vi "Actor Core.vi"(8 "error in":errorcluster, 11 "CS++DSCAlarmViewer in":refnum<class "CS++DSCAlarmViewer.lvclass">) -> (0 "error out":errorcluster, 3 "Actor out":refnum<class "Actor.lvclass">)   [LabVIEW 2013, in "CS++DSCAlarmViewer.lvlib" / "CS++DSCAlarmViewer.lvclass"]
doc: "(<B>Filename</B>: Actor Framework.lvlib:Actor.lvclass:Actor Core.vi)\n\nReceives messages to the actor, reacts to them, and initiates any error handling that may shut the actor down.\n\nDescendant classes may override this VI to append parallel tasks for the actor to complete while it handles messages. Overrides use the Call Parent Method node."
uses:
  CS++DSCAlarmViewer.lvclass
  <vilib>/ActorFramework/Actor/Actor.lvclass
  CS++DSCAlarmViewer.lvclass/CS++DSCAlarmViewer.ctl
  Core/Actors/CS++GUIActor/CS++GUIActor.lvclass/CS++GUIActor.ctl
  Core/Actors/CS++BaseActor/CS++BaseActor.lvclass/CS++BaseActor.ctl
  Core/Actors/CS++GUIActor/CS++GUIActor.lvclass
  <vilib>/ActorFramework/Actor/Actor.lvclass/Actor.ctl
  <vilib>/ActorFramework/Message Enqueuer/Message Enqueuer.lvclass/Message Enqueuer.ctl
  <vilib>/ActorFramework/Message Enqueuer/Init from Existing Queue.vi
  <vilib>/ActorFramework/Message Enqueuer/Enqueue.vi
  <vilib>/ActorFramework/Message Priority Queue/Priority Enqueue.vi
  <vilib>/ActorFramework/Message Enqueuer/Message Enqueuer.lvclass
  <vilib>/ActorFramework/Stop Msg/Stop Msg.lvclass
  Core/Actors/CS++BaseActor/CS++BaseActor.lvclass
panel:
  in  "Alarm and Event Display":refnum<k7>(container)
  in  "Stop Button":bool
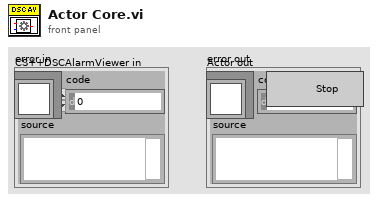
[diagram p1: front panel]
types:
  T1 = enum32{"Invalid", "Standard", "Closed", "Hidden", "Minimized", "Maximized"}
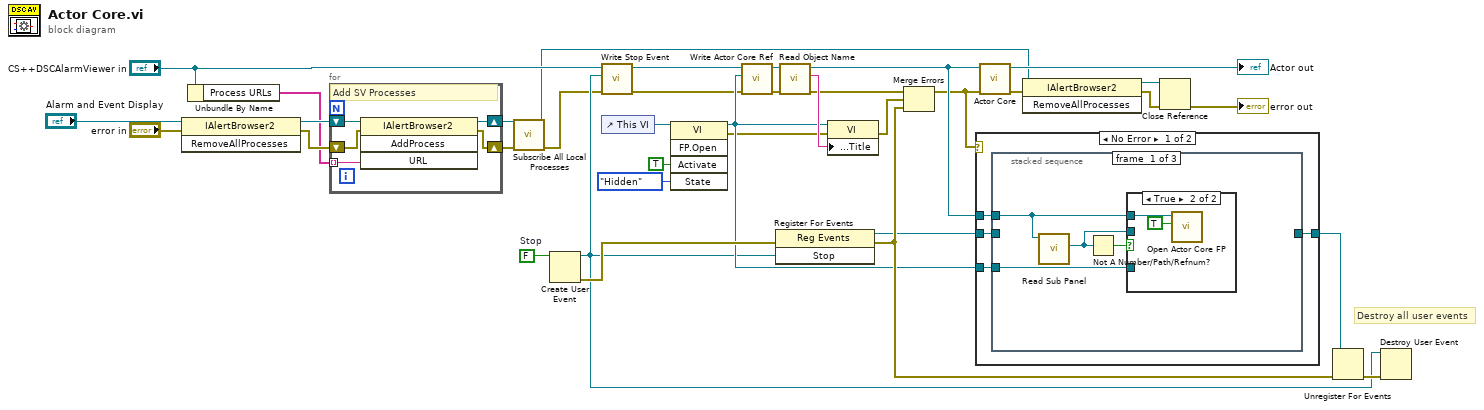
[diagram p0: block diagram]
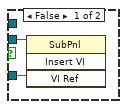
[diagram p2: hidden frame]
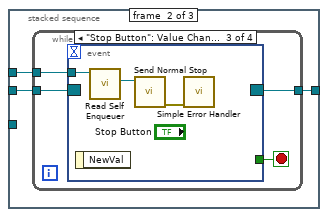
[diagram p3: hidden frame]
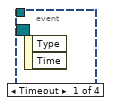
[diagram p4: hidden frame]
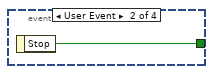
[diagram p5: hidden frame]
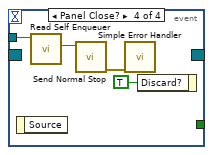
[diagram p6: hidden frame]
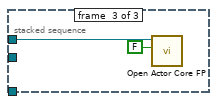
[diagram p7: hidden frame]
diagram:
  w31 = FALSE  # Stop
  # "Destroy all user events"
  n1 = invoke class="IAlertBrowser2" method="RemoveAllProcesses"(reference="Alarm and Event Display", error in="error in") -> (reference out=w14:refnum<k7>, error out=w12:errorcluster)  [unwired: 1 in, 1 out]
  n2 = Unbundle By Name("CS++DSCAlarmViewer in") -> ("Process URLs"=w9:string[])
  n3 = for {
    tunnel: w9 -> [w37] mode=indexing
    shift-right: [w40] -> w13
    shift-left: w14 -> [w41]
    shift-right: [w38] -> w11
    shift-left: w12 -> [w39]
    # "Add SV Processes"
    n4 = invoke class="IAlertBrowser2" method="AddProcess"(reference=w41, error in=w39, "URL"=w37) -> (reference out=w40:refnum<k7>, error out=w38:errorcluster)  [unwired: 1 in, 2 out]
  }
  n5 = call <vilib>:"Subscribe All Local Processes.vi"("error in"=w11, "Alarm & Event Displayer reference"=w13) -> ("error out"=w7:errorcluster, "Alarm & Event Displayer reference out"=w3:refnum<k7>)  [unwired: 8 in]
  n6 = Create User Event(user event datatype=w31) -> (user event=w22:refnum<user-event>, error out=w28:errorcluster)  [unwired: 1 in]
  n7 = call "Write Stop Event.vi"("error in (no error)"=w7, "Stop"=w22, "CS++GUIActor in"="CS++DSCAlarmViewer in") -> ("error out"=w20:errorcluster, "CS++GUIActor out"=w21:refnum<class "CS++DSCAlarmViewer.lvclass">)  [unwired: 7 in]
  n8 = control-ref of="This VI"() -> (w35:refnum<vi>)
  n9 = invoke class="VI" method="FP.Open"(reference=w35, "Activate"=TRUE ("Activate?"), "State"=T1."Hidden") -> (reference out=w24:refnum<vi>, error out=w23:errorcluster)  [unwired: 2 in, 3 out]
  n10 = call "Write Actor Core Ref.vi"("error in (no error)"=w20, "Actor Core Ref"=w24, "CS++BaseActor in"=w21) -> ("error out"=w19:errorcluster, "CS++BaseActor out"=w18:refnum<class "CS++DSCAlarmViewer.lvclass">)  [unwired: 7 in]
  n11 = register-events(error in=w28, w22) -> (reference out=w26:refnum<event-registration>, error out=w27:errorcluster)  [unwired: 1 in]
  n12 = call "Read Object Name.vi"("error in (no error)"=w19, "CS++BaseActor in"=w18) -> ("error out"=w17:errorcluster, "Object Name"=w32:string, "CS++BaseActor out"=w16:refnum<class "CS++DSCAlarmViewer.lvclass">)  [unwired: 7 in]
  n13 = property class="VI"(reference=w24, error in=w23, "Front Panel.Title"=w32) -> (error out=w30:errorcluster)  [unwired: 1 out]
  n14 = Merge Errors(w17, w30, w27) -> (w15:errorcluster)
  n15 = case shown="No Error" w15 {
    tunnel: w16 -> [w45 _]
    tunnel: w26 -> [w44 w71]
    tunnel: [w43 w71] -> w25
    tunnel: w24 -> [w42 _]
    frame No Error {
      n16 = stacked-sequence {
        tunnel: w45 -> [w47 w55 w70]
        tunnel: w44 -> [_ w56 _]
        tunnel: [_ w54 _] -> w43
        tunnel: w42 -> [w48 _ _]
        frame #0 {
          n17 = call "Read Sub Panel.vi"("CS++GUIActor in"=w47) -> ("Sub Panel"=w46:refnum<vi>)  [unwired: 8 in, 2 out]
          n18 = Not A Number/Path/Refnum?(number/path/refnum=w46) -> (NaN/Path/Refnum?=w49:bool)
          n19 = case shown="True" w49 {
            tunnel: w47 -> [_ w53]
            tunnel: w46 -> [w51 _]
            tunnel: w48 -> [w50 _]
            frame False {
              n20 = invoke class="SubPnl" method="Insert VI"(reference=w51, "VI Ref"=w50) -> ()  [unwired: 2 in, 4 out]
            }
            frame True {
              n21 = call "Open Actor Core FP.vi"("Open FP (F)"=TRUE, "CS++BaseActor in"=w53) -> ()  [unwired: 8 in, 2 out]
            }
          }
        }
        frame #1 {
          n22 = while {
            tunnel: w56 -> [w60]
            tunnel: w55 -> [w59]
            tunnel: [w57] -> w54
            stop <- w58 stop-if-true
            n23 = event shown="[2] \"Stop Button\": Value Change" {
              selector: w60 -> [_ _ _ _]
              dyn-events: [_ _ _ _] -> w57
              timeout: _ -> [_ _ _ _]
              tunnel: w59 -> [_ _ w64 w68]
              tunnel: [_ w61 _ _] -> w58
              event Timeout {
                n24 = event-data() -> ()  [unwired: 1 in, 2 out]
              }
              event User Event {
                n25 = event-data() -> ("Stop"=w61:bool)  [unwired: 1 in]
              }
              event "Stop Button": Value Change {
                n26 = event-data() -> ()  [unwired: 1 in, 1 out]
                n27 = call <vilib>:"Read Self Enqueuer.vi"("Actor"=w64) -> ("Self Enqueuer"=w63:refnum<class "Message Enqueuer.lvclass">)  [unwired: 10 in]
                n28 = call <vilib>:"Send Normal Stop.vi"("Message Enqueuer"=w63) -> ("error out"=w62:errorcluster)  [unwired: 10 in]
                n29 = call <vilib>:"Simple Error Handler.vi"("error in (no error)"=w62) -> ()  [unwired: 4 in, 5 out]
              }
              event Panel Close? {
                n30 = event-data() -> ()  [unwired: 1 in, 1 out]
                n31 = call <vilib>:"Read Self Enqueuer.vi"("Actor"=w68) -> ("Self Enqueuer"=w67:refnum<class "Message Enqueuer.lvclass">)  [unwired: 10 in]
                n32 = call <vilib>:"Send Normal Stop.vi"("Message Enqueuer"=w67) -> ("error out"=w66:errorcluster)  [unwired: 10 in]
                n33 = call <vilib>:"Simple Error Handler.vi"("error in (no error)"=w66) -> ()  [unwired: 4 in, 5 out]
                n34 = event-data("Discard?"=TRUE) -> ()  [unwired: 1 in, 1 out]
              }
            }
          }
        }
        frame #2 {
          n35 = call "Open Actor Core FP.vi"("Open FP (F)"=FALSE, "CS++BaseActor in"=w70) -> ()  [unwired: 8 in, 2 out]
        }
      }
    }
    frame Error {
    }
  }
  n36 = call-parent "Actor Core.vi"("error in"=w15, "CS++GUIActor in"=w16) -> ("error out"=w2:errorcluster, "Actor out"=→"Actor out":refnum<class "Actor.lvclass">)  [unwired: 8 in]
  n37 = invoke class="IAlertBrowser2" method="RemoveAllProcesses"(reference=w3, error in=w2) -> (reference out=w5:refnum<k7>, error out=w4:errorcluster)  [unwired: 1 in, 1 out]
  n38 = Close Reference(reference=w5, error in (no error)=w4) -> (error out=→"error out":errorcluster)
  n39 = Unregister For Events(event registration refnum=w25, error in=w27) -> (error out=w29:errorcluster)
  n40 = Destroy User Event(user event=w22, error in=w29) -> ()  [unwired: 1 out]
